vi "Rx Int Wait Event.vi"(9 "dwMilliseconds":u32, 10 "hEvt":u32, 11 "devId":i32) -> (1 "devId out":i32, 2 "hEvt out":u32, 3 "function return":u32)   [LabVIEW 2013, in "CHR34XXX.lvlib"]
doc: "DLL DWORD __stdcall CHR34XXX_RxInt_WaitEvent(IN int devId,IN HANDLE hEvt,IN DWORD dwMilliseconds);"
uses:
  CHR34XXX.lvlib
  CHR34XXX.dll
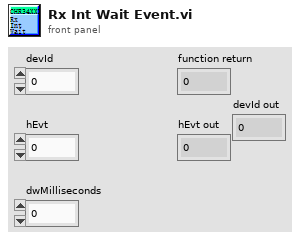
[diagram p1: front panel]
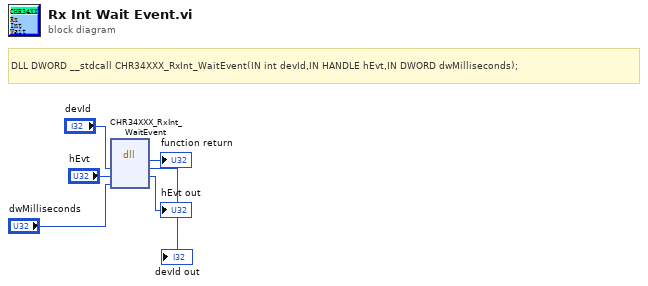
[diagram p0: block diagram]
diagram:
  # "DLL DWORD __stdcall CHR34XXX_RxInt_WaitEvent(IN int devId,IN HANDLE hEvt,IN DWORD dwMilliseconds);"
  n1 = dll-call lib="C:/Users/Administrator/Desktop/CHR34XXX_lv/lv_lib/CHR34XXX.*" fn="CHR34XXX_RxInt_WaitEvent"("devId"="devId", "hEvt"="hEvt", "dwMilliseconds"="dwMilliseconds") -> (→"function return":u32, "devId"=→"devId out":i32, "hEvt"=→"hEvt out":u32)  [unwired: 4 in, 2 out]
